vi "SCB RT.vi"() -> ()   [LabVIEW 2015]
uses:
  <vilib>/Platform/TimedLoop/XDataNode/XDataNode.xnode
  <vilib>/Platform/TimedLoop/XDataNode/nitl_modes.ctl
  <vilib>/Platform/TimedLoop/XDataNode/XDNodeRunTimeDep.lvlib
  <vilib>/Platform/TimedLoop/XDataNode/wakeup.ctl
  <vilib>/Platform/TimedLoop/XDataNode/timing_clust.ctl
  <vilib>/Platform/TimedLoop/XDataNode/loadnilvce.vi
  SC2 states.ctl
  <vilib>/Motion/BlockNode/FB.NIMotion.xnode
  <vilib>/nisyscfg/nisyscfg.lvlib
  Encoder bit cluster.ctl
  <vilib>/Motion/Express/_s/nimc.fb.straightLineMove.startStraightLineMove.axis.modeRelative.0.vi
  Horizontal Rod states.ctl
  GV states.ctl
  Vertical Rod states.ctl
  <vilib>/nisyscfg/Find Hardware.vi
  Bypass control.ctl
panel:
  out "SCB Wheel GV Bypass":bool
  out "SCB Sample Rod Bypass":bool
  out "SCB Retract Rod Bypass":bool
  out "SCB Ion Source GV Bypass":bool
  out "SCB Insert Rod Bypass":bool
  in  "Current State":T1
  out "Encoder displacement":i32
  in  "Random Sample":bool
  out "Within window?":bool
  in  "Stop":bool
  out "Motor status":bool=TRUE
  in  "Encoder offset":i32=-1277
  in  "Start Sample Change":bool
  out "SCB State Control":T1=enum."wait"
  out "Encoder readback":errorcluster
  in  "error in (no error)":errorcluster
  out "status":bool
  out "Encoder destination":i32
  in  "New Move (Motor steps)":dbl=10000.0 format="%#_13g"
  in  "New Sample":i16
  in  "Step Window radius":i32=2
  out "Converted Encoder":bool[](array[boolean])
  in  "Motion Resource":refnum<k21>="Axis SCB motor"
  out "Straight Line Move":errorcluster
  out "Raw Encoder":bool[](array[boolean])
  out "Encoder rotation":u16(graph)
  out "Encoder Position":i32
  # "Encoder offset required to \n\"line up\" encoder with wheel.\nSample 64 is -1021 encoder steps\n (or +15362 steps) from the \nencoder's zero point.. Note: Sample \nand encoder numbering run in \nopposite directions"
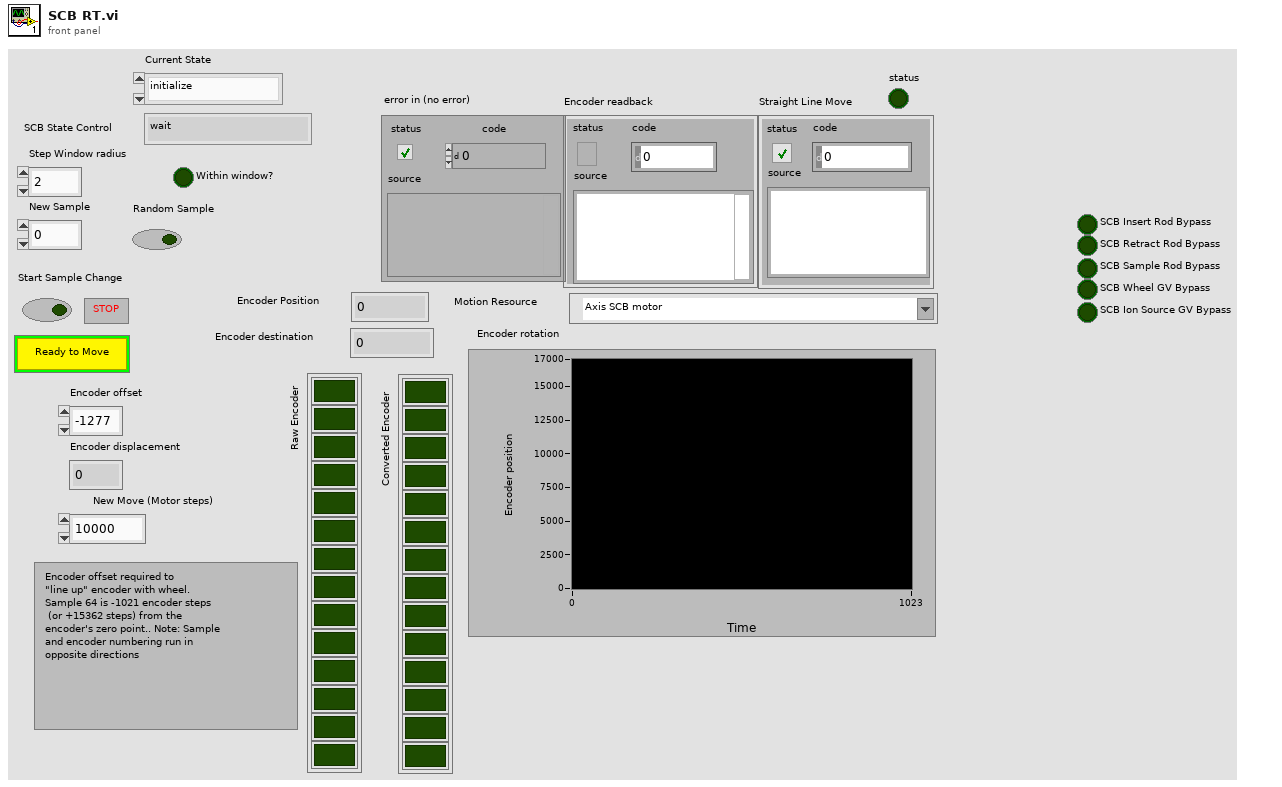
[diagram p1: front panel]
types:
  T1 = typedef "SC2 states.ctl" = enum16{"initialize", "wait", "change sample start", "change sample", "check position", "rotate wheel", "rotate complete", "sample rod up", "sample rod down", "retract rod in", "retract rod out", "insert rod in", "insert rod out", "bellows SC GV open", "bellows SC GV close", "bellows IS GV open", "bellows IS GV close", "vent source", "pump source", "rezero", "Shutdown"}
  T2 = typedef "XDNodeRunTimeDep.lvlib/timing_clust.ctl" = cluster{"Expected End [f-1]":u64, "Actual End [f-1]":u64, "Finished Late? [f-1]":bool, "Expected End [i-1]":u64, "Actual End [i-1]":u64, "Finished Late? [i-1]":bool, "Expected Start [i]":u64, "Actual Start [i]":u64, "Expected Start [f]":u64, "Actual Start [f]":u64, "Source Name":string, "Structure Name":string, "Period":i64, "Deadline":i64, "Offset":i64, "Start":i64, "Priority":i32, "Timeout":i32, "Mode":T3, "Wakeup Reason":T4, "Error":errorcluster, "Source Type":string, "Secondary Source Type":string, "Global End Time":u64, "Global Start Time":u64, "Frame Duration":u64, "Iteration Duration":u64, "Assigned CPU":i32, "I/O Scan Engine Mode":u32}
  T3 = typedef "XDNodeRunTimeDep.lvlib/nitl_modes.ctl" = enum32{"No Change", "Process missed periods, maintain original phase", "Discard missed periods, maintain original phase", "Process missed periods, ignore original phase", "Discard missed periods, ignore original phase"}
  T4 = typedef "XDNodeRunTimeDep.lvlib/wakeup.ctl" = enum32{"Normal", "Aborted", "Asynchronous wakeup", "Timing source error", "Timed loop error", "Timeout"}
  T5 = typedef "GV states.ctl" = enum16{"status unclear", "closed", "open"}
  T6 = typedef "Vertical Rod states.ctl" = enum16{"status unclear", "rod down", "rod up"}
  T7 = typedef "Horizontal Rod states.ctl" = enum16{"status unclear", "rod in", "rod out"}
  T8 = cluster{"Sample Rod":u16, "Insert Rod":u16, "Retract Rod":u16, "Wheel GV":u16, "Ion Source GV":u16, "Rotate Wheel":u16}
  T9 = typedef "Encoder bit cluster.ctl" = cluster{"MSB":bool, "13th bit":bool, "12th bit":bool, "11th bit":bool, "10th bit":bool, "9th bit":bool, "8th bit":bool, "7th bit":bool, "6th bit":bool, "5th bit":bool, "4th bit":bool, "3rd bit":bool, "2nd bit":bool, "LSB":bool}
  T10 = typedef "Bypass control.ctl" = cluster{"SCB Insert Rod Bypass":bool, "SCB Ion Source GV Bypass":bool, "SCB Retract Rod Bypass":bool, "SCB Sample Rod Bypass":bool, "SCB Wheel GV Bypass":bool}
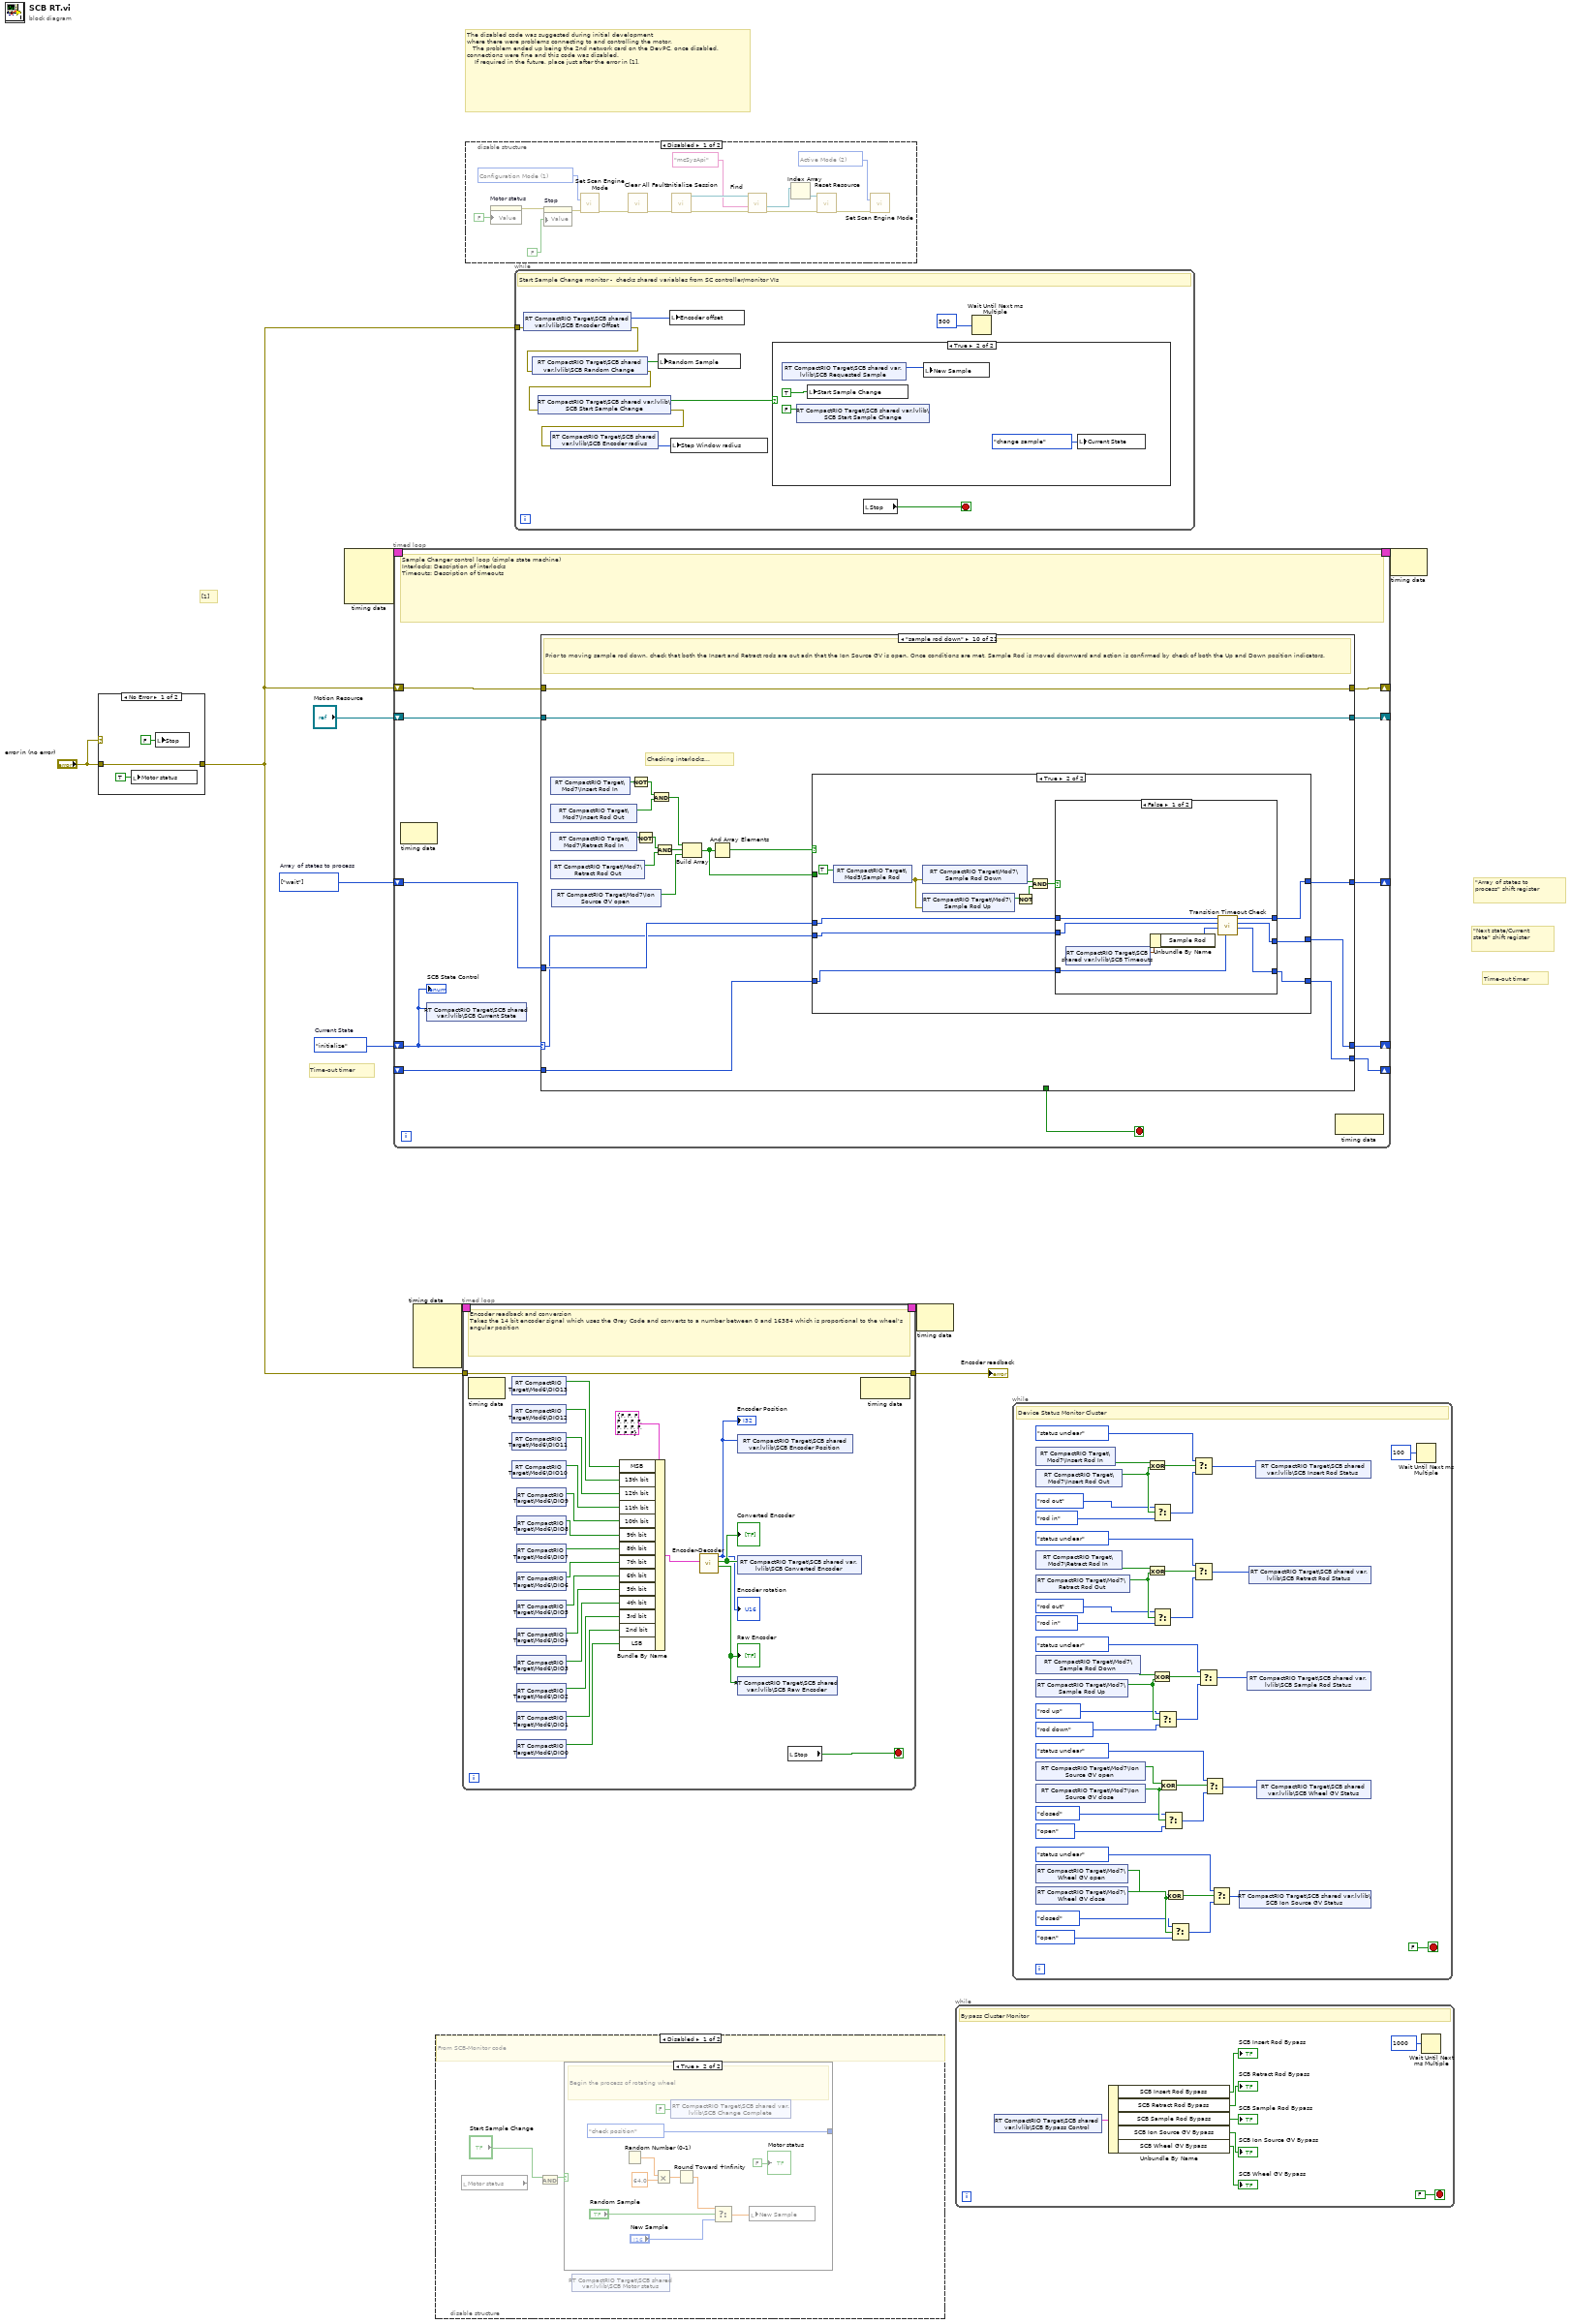
[diagram p0: block diagram]
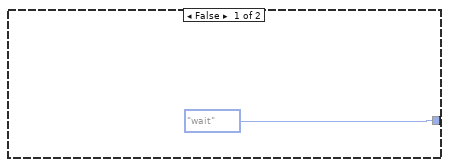
[diagram p2: hidden frame]
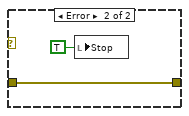
[diagram p4: hidden frame]
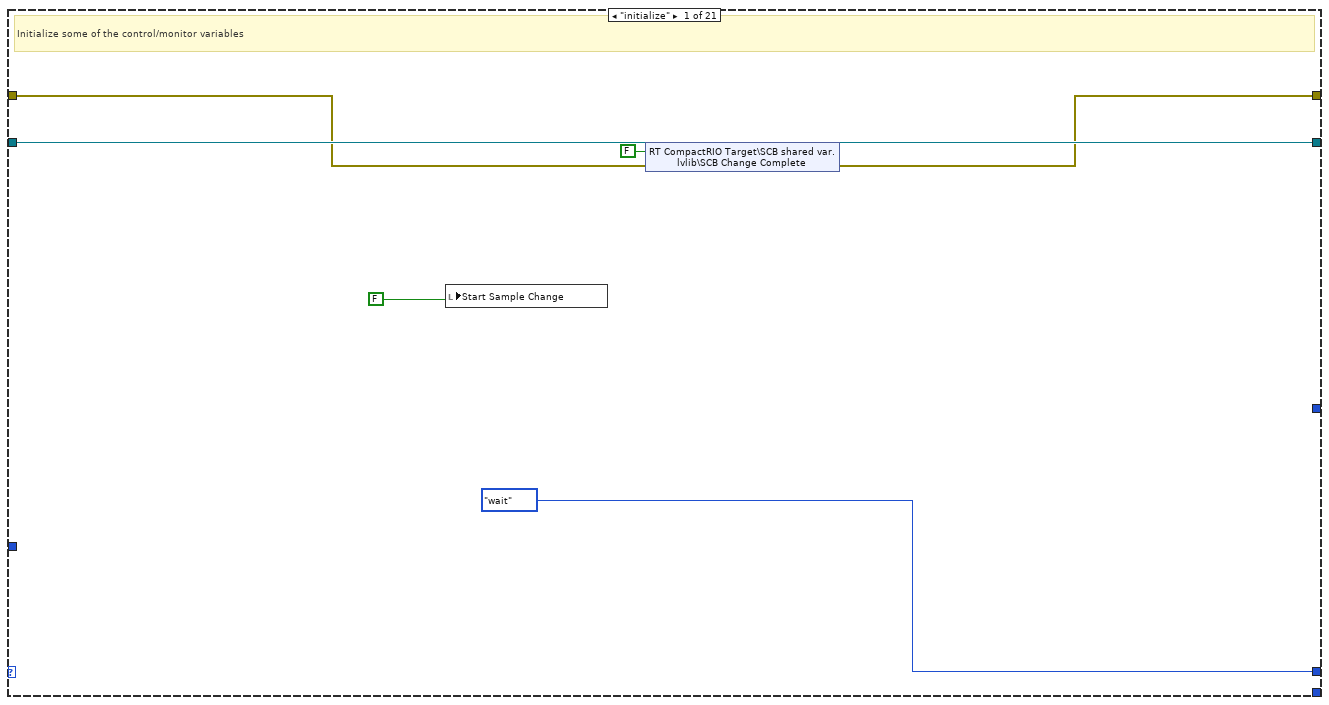
[diagram p7: hidden frame]
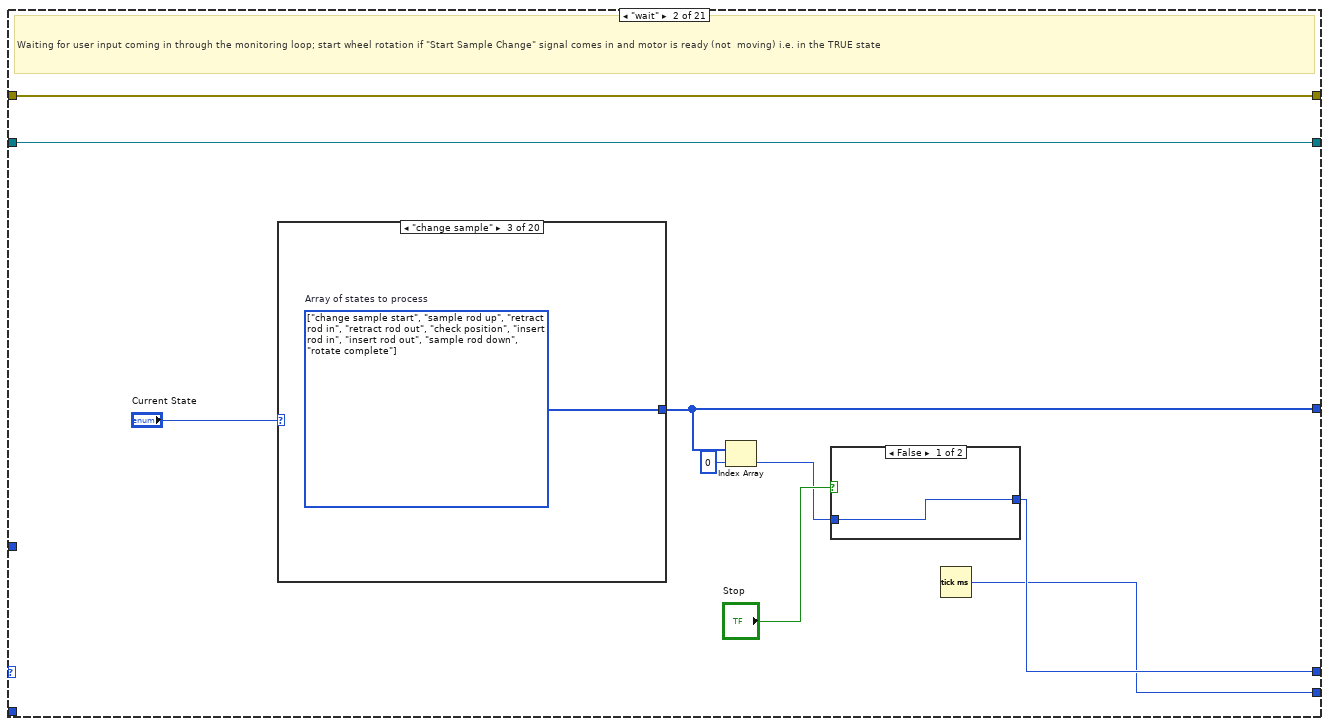
[diagram p8: hidden frame]
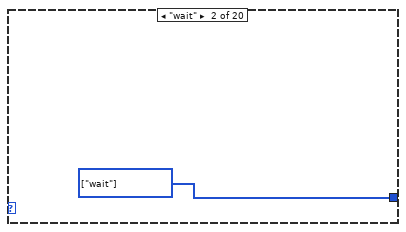
[diagram p10: hidden frame]
diagram:
  w1 = T1[] [enum."wait"] items=["initialize", "wait", "change sample start", "change sample", "check position", "rotate wheel", "rotate complete", "sample rod up", "sample rod down", "retract rod in", "retract rod out", "insert rod in", "insert rod out", "bellows SC GV open", "bellows SC GV close", "bellows IS GV open", "bellows IS GV close", "vent source", "pump source", "rezero", "Shutdown"]  # Array of states to process
  w5 = SC2_states."initialize"  # Current State
  # "Time-out timer"
  # "Time-out timer"
  # "\"Next state/Current\nstate\" shift register"
  # "\"Array of states to \nprocess\" shift register"
  # "[1]"
  # "The disabled code was suggested during initial development\nwhere there were problems connecting to and controlling the motor.\n   The problem ended up being the 2nd network card on the DevPC, once disabled, connections were fine and this code was disabled.  \n    If required in the future, place just after the error in [1]."
  n1 = case shown="No Error" "error in (no error)" {
    tunnel: "error in (no error)" -> [w12 w15]
    tunnel: [w12 w15] -> w3
    frame No Error {
      n2 = local write "Motor status"(TRUE ("Motor status")) -> ()
      n3 = local write "Stop"(FALSE ("Stop")) -> ()
    }
    frame Error {
      n4 = local write "Stop"(TRUE ("Stop")) -> ()
    }
  }
  n5 = node-c288() -> (w8:T2)  [unwired: 4 in]
  n6 = timed-loop {
    timing: w8 -> [_]
    timing-out: [_] -> w7
    shift-right: [w25] -> _
    shift-left: w5 -> [w22]
    shift-right: [w24] -> _
    shift-left: "Motion Resource" -> [w26]
    shift-right: [w20] -> _
    shift-left: w1 -> [w19]
    shift-right: [w18] -> _
    shift-left: _ -> [w17]
    shift-right: [w16] -> _
    shift-left: w3 -> [w23]
    stop <- w21 stop-if-true
    # "Sample Changer control loop (simple state machine)\nInterlocks: Description of interlocks\nTimeouts: Description of timeouts"
    n7 = node-c288() -> ()  [unwired: 1 in, 1 out]
    n8 = shared-variable "RT CompactRIO Target\\SCB shared var.lvlib\\SCB Current State"(w22) -> ()  [unwired: 1 in, 1 out]
    n9 = case shown="\"sample rod down\"" w22 {
      selector: w22 -> [_ _ w55 _ _ _ _ _ w140 w164 w229 w304 _ w335 _ w363 _ w421 _ _ _]
      tunnel: w26 -> [w31 w41 w46 w61 w89 w114 w134 _ _ w160 w240 _ _ w327 _ _ _ w416 _ _ _]
      tunnel: [SC2_states."wait" w39 w51 w74 w84 SC2_states."wait" SC2_states."Shutdown" _ w138 w165 w243 w300 _ w332 _ w361 _ w418 _ _ _] -> w25
      tunnel: [w31 w41 w46 w61 w81 w111 w134 _ _ w160 w240 _ _ w327 _ _ _ w416 _ _ _] -> w24
      tunnel: w23 -> [w28 w33 w49 w58 w78 _ _ _ _ w161 w241 _ _ w328 _ _ _ w415 _ _ _]
      tunnel: [_ _ _ _ _ _ TRUE _ _ _ _ _ _ _ _ _ _ _ _ _ _] -> w21
      tunnel: [_ w37 w54 _ w75 _ _ _ w139 w166 w244 w301 _ w333 _ w362 _ w417 _ _ _] -> w20
      tunnel: w19 -> [_ _ w56 _ w75 _ _ _ w141 w167 w228 w302 _ w336 _ w364 _ w422 _ _ _]
      tunnel: [_ w34 w50 w57 _ _ _ _ w137 w162 w242 w299 _ w331 _ w360 _ w419 _ _ _] -> w18
      tunnel: w17 -> [_ _ _ _ _ _ _ _ w136 w163 w245 w303 _ w334 _ w359 _ w420 _ _ _]
      tunnel: [w27 w33 w47 w58 w76 _ _ _ _ w161 w241 _ _ w328 _ _ _ w415 _ _ _] -> w16
      frame "initialize" {
        # "Initialize some of the control/monitor variables"
        n10 = local write "Start Sample Change"(FALSE ("Start Sample Change")) -> ()
        n11 = shared-variable "RT CompactRIO Target\\SCB shared var.lvlib\\SCB Change Complete"(FALSE ("SC2 Change Complete"), error in=w28) -> (error out=w27:errorcluster)
      }
      frame "wait" {
        # "Waiting for user input coming in through the monitoring loop; start wheel rotation if \"Start Sample Change\" signal comes in and motor is ready (not  moving) i.e. in the TRUE state"
        n12 = case shown="\"change sample\"" "Current State" {
          tunnel: [_ w42 w43 _ _ _ _ _ _ _ _ _ _ _ _ _ _ _ _ _] -> w37
          frame "initialize", Default {
          }
          frame "wait" {
            w42 = T1[] [enum."wait"] items=["initialize", "wait", "change sample start", "change sample", "check position", "rotate wheel", "rotate complete", "sample rod up", "sample rod down", "retract rod in", "retract rod out", "insert rod in", "insert rod out", "bellows SC GV open", "bellows SC GV close", "bellows IS GV open", "bellows IS GV close", "vent source", "pump source", "rezero", "Shutdown"] ("Array of states to process")
          }
          frame "change sample" {
            w43 = T1[] [enum."change sample start", enum."sample rod up", enum."retract rod in", enum."retract rod out", enum."check position", enum."insert rod in", enum."insert rod out", enum."sample rod down", enum."rotate complete"] items=["initialize", "wait", "change sample start", "change sample", "check position", "rotate wheel", "rotate complete", "sample rod up", "sample rod down", "retract rod in", "retract rod out", "insert rod in", "insert rod out", "bellows SC GV open", "bellows SC GV close", "bellows IS GV open", "bellows IS GV close", "vent source", "pump source", "rezero", "Shutdown"]  # Array of states to process
          }
          frame "check position" {
          }
          frame "rotate wheel" {
          }
          frame "rotate complete" {
          }
          frame "sample rod up" {
          }
          frame "sample rod down" {
          }
          frame "retract rod in" {
          }
          frame "retract rod out" {
          }
          frame "insert rod in" {
          }
          frame "insert rod out" {
          }
          frame "bellows SC GV open" {
          }
          frame "bellows SC GV close" {
          }
          frame "bellows IS GV open" {
          }
          frame "bellows IS GV close" {
          }
          frame "vent source" {
          }
          frame "pump source" {
          }
          frame "rezero" {
          }
          frame "Shutdown" {
          }
        }
        n13 = Index Array(array=w37, index=0) -> (element=w36:T1)
        n14 = case shown="False" "Stop" {
          tunnel: [w44 SC2_states."Shutdown"] -> w39
          tunnel: w36 -> [w44 _]
          frame False {
          }
          frame True {
          }
        }
        n15 = Tick Count (ms)() -> (millisecond timer value=w34:u32)
      }
      frame "change sample start" {
        n16 = call "Modify array of states.vi"("Current State"=w55, "Array of states to process"=w56) -> ("Next State"=w51:T1, "Modified Array of states"=w54:T1[])  [unwired: 8 in]
        n17 = shared-variable "RT CompactRIO Target\\SCB shared var.lvlib\\SCB Change Complete"(FALSE ("SCB Change Complete"), error in=w49) -> (error out=w48:errorcluster)
        n18 = shared-variable "RT CompactRIO Target\\SCB shared var.lvlib\\SCB Changing Sample"(TRUE ("SCB Changing Sample"), error in=w48) -> (error out=w47:errorcluster)
        n19 = Tick Count (ms)() -> (millisecond timer value=w50:u32)
      }
      frame "check position" {
        # "Number of steps for\nmotor to move"
        # "number of encoder steps to progress"
        # "14-bit encoder has 2^14 steps/rev"
        # "Motor steps per revolution"
        # "In this case, the wheel's position is checked and if it's within the Step WIndow Radius of the desired position, the state machine progresses to the \"rotate complete\" state.  If not, the number of encoder steps to progress to the desired position is stepped through by going to the \"rotate wheel\" state"
        n20 = local read "Encoder Position"() -> (w68:i32)
        n21 = local read "New Sample"() -> (w60:i16)
        n22 = call "Sample-Encoder conversion.vi"("Encoder Position"=w68, "Step Window radius"="Step Window radius", "New Sample Number"=w60, "Encoder offset"="Encoder offset") -> ("Encoder destination"=w66:i32, "Within Range?"=w59:bool, "Encoder displacement"=w69:i32)  [unwired: 5 in]
        "Encoder destination" <- w66
        "Within window?" <- w59
        "Encoder displacement" <- w69
        n23 = shared-variable "RT CompactRIO Target\\SCB shared var.lvlib\\SCB Encoder destination"(w66) -> ()  [unwired: 1 in, 1 out]
        n24 = Divide(x=50000.0, y=16384.0) -> (x/y=w73:dbl)
        n25 = Multiply(x=w73, y=w69) -> (x*y=w70:dbl)
        n26 = local write "Motor status"(w59) -> ()
        n27 = shared-variable "RT CompactRIO Target\\SCB shared var.lvlib\\SCB Motor status"(w59) -> ()  [unwired: 1 in, 1 out]
        n28 = Round To Nearest(number=w70) -> (nearest integer value=w63:dbl)
        n29 = local write "New Move (Motor steps)"(w63) -> ()
        n30 = Select(t=SC2_states."rotate complete", s=w59, f=SC2_states."rotate wheel") -> (s? t:f=w74:T1)
        n31 = Tick Count (ms)() -> (millisecond timer value=w57:u32)
      }
      frame "rotate wheel" {
        w90 = 10000.0
        # "Prior to Rotating Wheel, both Insert and Retract rods' positions are checked.  Once confirmed, step motor to progress though New Move number of steps and then returns to \"check position\" to determine that the move was successful"
        n32 = local read "Start Sample Change"() -> (w85:bool)
        n33 = Multiply(x="New Move (Motor steps)", y=-1.0) -> (x*y=w80:dbl)
        n34 = xnode "Straight-Line Move\n(Relative)"("error in"=w78, "resource"=w89, "execute"=w85, "position"=w80, "velocity"=w90, "acceleration"=w90) -> ("error out"=w76:errorcluster, "resource out"=w81:refnum<k21>, "done"=w82:bool)
        "Straight Line Move" <- w76
        n35 = Unbundle By Name(w76) -> ("status"=→"status":bool)
        n36 = Not(x=w82) -> (.not. x?=w77:bool)
        n37 = local write "Start Sample Change"(w77) -> ()
        n38 = Select(t=SC2_states."check position", s=w82, f=SC2_states."rotate wheel") -> (s? t:f=w84:T1)
      }
      frame "rotate complete" {
        # "Stop SLM; set monitor variables"
        n39 = local read "New Sample"() -> (w109:i16)
        n40 = xnode "Straight-Line Move\n(Relative)"("resource"=w114, "execute"=FALSE) -> ("resource out"=w111:refnum<k21>)  [unwired: 4 in, 2 out]
        n41 = shared-variable "RT CompactRIO Target\\SCB shared var.lvlib\\SCB Current Sample"(w109) -> ()  [unwired: 1 in, 1 out]
        n42 = shared-variable "RT CompactRIO Target\\SCB shared var.lvlib\\SCB Change Complete"(TRUE ("SC2 Change Complete")) -> ()  [unwired: 1 in, 1 out]
        n43 = local write "Start Sample Change"(FALSE ("Start Sample Change")) -> ()
      }
      frame "Shutdown" {
      }
      frame "change sample" {
      }
      frame "sample rod up" {
        # "Move Sample Rod upward; check both the up and down position indicators"
        n44 = shared-variable "RT CompactRIO Target\\Mod5\\Sample Rod"(FALSE) -> (error out=w135:errorcluster)  [unwired: 1 in]
        n45 = shared-variable "RT CompactRIO Target\\Mod7\\Sample Rod Up"(error in=w135) -> (w143:bool)  [unwired: 1 out]
        n46 = shared-variable "RT CompactRIO Target\\Mod7\\Sample Rod Down"(error in=w135) -> (w145:bool)  [unwired: 1 out]
        n47 = Not(x=w145) -> (.not. x?=w144:bool)
        n48 = And(x=w143, y=w144) -> (x .and. y?=w142:bool)
        n49 = case shown="True" w142 {
          tunnel: w141 -> [w152 w159]
          tunnel: w140 -> [w154 w158]
          tunnel: [w151 w157] -> w139
          tunnel: [w153 w156] -> w138
          tunnel: [w149 w155] -> w137
          tunnel: w136 -> [w150 _]
          frame False {
            # "Sample rod is not up. Check to see if timeout limit has been reached"
            n50 = shared-variable "RT CompactRIO Target\\SCB shared var.lvlib\\SCB Timeouts"() -> (w148:T8)  [unwired: 1 in, 1 out]
            n51 = Unbundle By Name(w148) -> ("Sample Rod"=w147:u16)
            n52 = call "Transition Timeout Check.vi"("Start Time"=w150, "Timeout limit"=w147, "Current State in"=w154, "Modified Array of states in"=w152) -> ("millisecond timer value out"=w149:u32, "Next State"=w153:T1, "Modified Array of states out"=w151:T1[])  [unwired: 4 in, 1 out]
          }
          frame True {
            # "Sample Rod is up; progress to next state and reset timer."
            n53 = call "Modify array of states.vi"("Current State"=w158, "Array of states to process"=w159) -> ("Next State"=w156:T1, "Modified Array of states"=w157:T1[])  [unwired: 8 in]
            n54 = Tick Count (ms)() -> (millisecond timer value=w155:u32)
          }
        }
      }
      frame "sample rod down" {
        # "Checking interlocks..."
        # "Prior to moving sample rod down, check that both the Insert and Retract rods are out adn that the Ion Source GV is open. Once conditions are met, Sample Rod is moved downward and action is confirmed by check of both the Up and Down position indicators."
        n55 = shared-variable "RT CompactRIO Target\\Mod7\\Insert Rod In"() -> (w178:bool)  [unwired: 1 in, 1 out]
        n56 = shared-variable "RT CompactRIO Target\\Mod7\\Insert Rod Out"() -> (w175:bool)  [unwired: 1 in, 1 out]
        n57 = shared-variable "RT CompactRIO Target\\Mod7\\Retract Rod In"() -> (w177:bool)  [unwired: 1 in, 1 out]
        n58 = shared-variable "RT CompactRIO Target\\Mod7\\Retract Rod Out"() -> (w173:bool)  [unwired: 1 in, 1 out]
        n59 = shared-variable "RT CompactRIO Target\\Mod7\\Ion Source GV open"() -> (w171:bool)  [unwired: 1 in, 1 out]
        n60 = Not(x=w178) -> (.not. x?=w176:bool)
        n61 = Not(x=w177) -> (.not. x?=w174:bool)
        n62 = And(x=w176, y=w175) -> (x .and. y?=w170:bool)
        n63 = And(x=w174, y=w173) -> (x .and. y?=w172:bool)
        n64 = Build Array(w170, w172, w171) -> (w168:bool[])
        n65 = And Array Elements(Boolean array=w168) -> (logical AND=w169:bool)
        n66 = case shown="True" w169 {
          tunnel: w168 -> [w185 _]
          tunnel: w167 -> [w182 w203]
          tunnel: [w181 w200] -> w166
          tunnel: [w180 w199] -> w165
          tunnel: w164 -> [_ w202]
          tunnel: w163 -> [_ w201]
          tunnel: [w179 w198] -> w162
          frame False {
            n67 = Search 1D Array(1D array=w185, element=FALSE) -> (index of element=w183:i32)  [unwired: 1 in]
            n68 = case shown="2" w183 {
              tunnel: w182 -> [w188 w190 w196]
              tunnel: [w187 w191 w194] -> w181
              tunnel: [w186 w192 w195] -> w180
              frame 0, Default {
                w186 = SC2_states."insert rod out"
                # "Insert Rod not completely out"
                n69 = Insert Into Array(array=w188, index=0, new element=w186) -> (w187:T1[])
              }
              frame 1 {
                w192 = SC2_states."retract rod out"
                # "Retract Rod not completely out"
                n70 = Insert Into Array(array=w190, index=0, new element=w192) -> (w191:T1[])
              }
              frame 2 {
                w195 = SC2_states."bellows IS GV open"
                # "Ion Source GV is still closed"
                n71 = Insert Into Array(array=w196, index=0, new element=w195) -> (w194:T1[])
              }
            }
            n72 = Tick Count (ms)() -> (millisecond timer value=w179:u32)
          }
          frame True {
            n73 = shared-variable "RT CompactRIO Target\\Mod5\\Sample Rod"(TRUE ("Wheel GV")) -> (error out=w208:errorcluster)  [unwired: 1 in]
            n74 = shared-variable "RT CompactRIO Target\\Mod7\\Sample Rod Down"(error in=w208) -> (w205:bool)  [unwired: 1 out]
            n75 = shared-variable "RT CompactRIO Target\\Mod7\\Sample Rod Up"(error in=w208) -> (w207:bool)  [unwired: 1 out]
            n76 = Not(x=w207) -> (.not. x?=w206:bool)
            n77 = And(x=w205, y=w206) -> (x .and. y?=w204:bool)
            n78 = case shown="False" w204 {
              tunnel: w203 -> [w216 w222]
              tunnel: w202 -> [w215 w221]
              tunnel: [w210 w220] -> w200
              tunnel: [w211 w219] -> w199
              tunnel: [w212 w218] -> w198
              tunnel: w201 -> [w213 _]
              frame False {
                n79 = shared-variable "RT CompactRIO Target\\SCB shared var.lvlib\\SCB Timeouts"() -> (w217:T8)  [unwired: 1 in, 1 out]
                n80 = Unbundle By Name(w217) -> ("Sample Rod"=w214:u16)
                n81 = call "Transition Timeout Check.vi"("Start Time"=w213, "Timeout limit"=w214, "Current State in"=w215, "Modified Array of states in"=w216) -> ("millisecond timer value out"=w212:u32, "Next State"=w211:T1, "Modified Array of states out"=w210:T1[])  [unwired: 4 in, 1 out]
              }
              frame True {
                n82 = call "Modify array of states.vi"("Current State"=w221, "Array of states to process"=w222) -> ("Next State"=w219:T1, "Modified Array of states"=w220:T1[])  [unwired: 8 in]
                n83 = Tick Count (ms)() -> (millisecond timer value=w218:u32)
              }
            }
          }
        }
      }
      frame "retract rod in" {
        # "Checking interlocks..."
        # "Prior to moving Retract Rod inward, check that: (1) the Sample Rod is UP; (2) the Insert Rod is OUT; and (3) the Wheel GV is open. Once conditions are met, Retract Rod is moved inward and action is confirmed by check of both the IN and OUT position indicators."
        n84 = local read "SCB Insert Rod Bypass"() -> (w236:bool)
        n85 = shared-variable "RT CompactRIO Target\\SCB shared var.lvlib\\SCB Insert Rod Status"() -> (w238:T7)  [unwired: 1 in, 1 out]
        n86 = local read "SCB Sample Rod Bypass"() -> (w232:bool)
        n87 = shared-variable "RT CompactRIO Target\\SCB shared var.lvlib\\SCB Sample Rod Status"() -> (w231:T6)  [unwired: 1 in, 1 out]
        n88 = local read "SCB Wheel GV Bypass"() -> (w226:bool)
        n89 = shared-variable "RT CompactRIO Target\\SCB shared var.lvlib\\SCB Wheel GV Status"() -> (w224:T5)  [unwired: 1 in, 1 out]
        n90 = Equal?(x=w224, y=GV_states."open") -> (x = y?=w225:bool)
        n91 = Equal?(x=w231, y=Vertical_Rod_states."rod up") -> (x = y?=w233:bool)
        n92 = Equal?(x=w238, y=Horizontal_Rod_states."rod out") -> (x = y?=w237:bool)
        n93 = Or(x=w226, y=w225) -> (x .or. y?=w227:bool)
        n94 = Or(x=w232, y=w233) -> (x .or. y?=w234:bool)
        n95 = Or(x=w236, y=w237) -> (x .or. y?=w235:bool)
        n96 = Build Array(w235, w234, w227) -> (w246:bool[])
        n97 = And Array Elements(Boolean array=w246) -> (logical AND=w247:bool)
        n98 = case shown="False" w247 {
          tunnel: w246 -> [w254 _]
          tunnel: w228 -> [w251 w274]
          tunnel: [w250 w271] -> w244
          tunnel: [w249 w270] -> w243
          tunnel: w229 -> [_ w273]
          tunnel: w245 -> [_ w272]
          tunnel: [w248 w269] -> w242
          frame False {
            n99 = Search 1D Array(1D array=w254, element=FALSE) -> (index of element=w252:i32)  [unwired: 1 in]
            n100 = case shown="1" w252 {
              tunnel: w251 -> [w257 w259 w265]
              tunnel: [w256 w260 w263] -> w250
              tunnel: [w255 w261 w264] -> w249
              frame 0, Default {
                w255 = SC2_states."insert rod out"
                # "Insert Rod not completely out"
                n101 = Insert Into Array(array=w257, index=0, new element=w255) -> (w256:T1[])
              }
              frame 1 {
                w261 = SC2_states."sample rod up"
                # "Sample Rod not completely up"
                n102 = Insert Into Array(array=w259, index=0, new element=w261) -> (w260:T1[])
              }
              frame 2 {
                w264 = SC2_states."bellows SC GV open"
                # "Wheel GV is still closed"
                n103 = Insert Into Array(array=w265, index=0, new element=w264) -> (w263:T1[])
              }
            }
            n104 = Tick Count (ms)() -> (millisecond timer value=w248:u32)
          }
          frame True {
            n105 = shared-variable "RT CompactRIO Target\\Mod5\\Retract Rod"(TRUE ("Wheel GV")) -> (error out=w267:errorcluster)  [unwired: 1 in]
            n106 = shared-variable "RT CompactRIO Target\\SCB shared var.lvlib\\SCB Retract Rod Status"(error in=w267) -> (w268:T7)  [unwired: 1 out]
            n107 = case shown="\"rod in\"" w268 {
              tunnel: w274 -> [w282 w290 w296]
              tunnel: w273 -> [w281 w289 w295]
              tunnel: [w276 w284 w294] -> w271
              tunnel: [w277 w285 w293] -> w270
              tunnel: [w278 w286 w292] -> w269
              tunnel: w272 -> [w279 w287 _]
              frame "status unclear", Default {
                n108 = shared-variable "RT CompactRIO Target\\SCB shared var.lvlib\\SCB Timeouts"() -> (w283:T8)  [unwired: 1 in, 1 out]
                n109 = Unbundle By Name(w283) -> ("Retract Rod"=w280:u16)
                n110 = call "Transition Timeout Check.vi"("Start Time"=w279, "Timeout limit"=w280, "Current State in"=w281, "Modified Array of states in"=w282) -> ("millisecond timer value out"=w278:u32, "Next State"=w277:T1, "Modified Array of states out"=w276:T1[])  [unwired: 4 in, 1 out]
              }
              frame "rod out" {
                n111 = shared-variable "RT CompactRIO Target\\SCB shared var.lvlib\\SCB Timeouts"() -> (w291:T8)  [unwired: 1 in, 1 out]
                n112 = Unbundle By Name(w291) -> ("Retract Rod"=w288:u16)
                n113 = call "Transition Timeout Check.vi"("Start Time"=w287, "Timeout limit"=w288, "Current State in"=w289, "Modified Array of states in"=w290) -> ("millisecond timer value out"=w286:u32, "Next State"=w285:T1, "Modified Array of states out"=w284:T1[])  [unwired: 4 in, 1 out]
              }
              frame "rod in" {
                n114 = call "Modify array of states.vi"("Current State"=w295, "Array of states to process"=w296) -> ("Next State"=w293:T1, "Modified Array of states"=w294:T1[])  [unwired: 8 in]
                n115 = Tick Count (ms)() -> (millisecond timer value=w292:u32)
              }
            }
          }
        }
      }
      frame "retract rod out" {
        # "Move Retract Rod outward; check both the in and out position indicators"
        n116 = shared-variable "RT CompactRIO Target\\Mod5\\Retract Rod"(FALSE) -> (error out=w298:errorcluster)  [unwired: 1 in]
        n117 = shared-variable "RT CompactRIO Target\\SCB shared var.lvlib\\SCB Retract Rod Status"(error in=w298) -> (w297:T7)  [unwired: 1 out]
        n118 = case shown="\"rod out\"" w297 {
          tunnel: w302 -> [w311 w318 w324]
          tunnel: w304 -> [w313 w317 w326]
          tunnel: [w310 w316 w323] -> w301
          tunnel: [w312 w315 w325] -> w300
          tunnel: [w308 w314 w321] -> w299
          tunnel: w303 -> [w309 _ w322]
          frame "status unclear", Default {
            # "Retract rod is not out. Check to see if timeout limit has been reached"
            n119 = shared-variable "RT CompactRIO Target\\SCB shared var.lvlib\\SCB Timeouts"() -> (w307:T8)  [unwired: 1 in, 1 out]
            n120 = Unbundle By Name(w307) -> ("Retract Rod"=w306:u16)
            n121 = call "Transition Timeout Check.vi"("Start Time"=w309, "Timeout limit"=w306, "Current State in"=w313, "Modified Array of states in"=w311) -> ("millisecond timer value out"=w308:u32, "Next State"=w312:T1, "Modified Array of states out"=w310:T1[])  [unwired: 4 in, 1 out]
          }
          frame "rod out" {
            # "Retract Rod is out; progress to next state and reset timer."
            n122 = call "Modify array of states.vi"("Current State"=w317, "Array of states to process"=w318) -> ("Next State"=w315:T1, "Modified Array of states"=w316:T1[])  [unwired: 8 in]
            n123 = Tick Count (ms)() -> (millisecond timer value=w314:u32)
          }
          frame "rod in" {
            # "Retract rod is not out. Check to see if timeout limit has been reached"
            n124 = shared-variable "RT CompactRIO Target\\SCB shared var.lvlib\\SCB Timeouts"() -> (w320:T8)  [unwired: 1 in, 1 out]
            n125 = Unbundle By Name(w320) -> ("Retract Rod"=w319:u16)
            n126 = call "Transition Timeout Check.vi"("Start Time"=w322, "Timeout limit"=w319, "Current State in"=w326, "Modified Array of states in"=w324) -> ("millisecond timer value out"=w321:u32, "Next State"=w325:T1, "Modified Array of states out"=w323:T1[])  [unwired: 4 in, 1 out]
          }
        }
      }
      frame "insert rod in" {
        # "Prior to moving Insert Rod inward, check that: (1) the Sample Rod is UP; (2) the Retract Rod is OUT; and (3) the Wheel GV is open. Once conditions are met, Insert Rod is moved inward and action is confirmed by check of both the IN and OUT position indicators."
      }
      frame "insert rod out" {
        # "Move Insert Rod outward; check both the in and out position indicators"
        n127 = shared-variable "RT CompactRIO Target\\Mod5\\Insert Rod"(FALSE) -> (error out=w329:errorcluster)  [unwired: 1 in]
        n128 = shared-variable "RT CompactRIO Target\\SCB shared var.lvlib\\SCB Insert Rod Status"(error in=w329) -> (w330:T7)  [unwired: 1 out]
        n129 = case shown="\"rod out\"" w330 {
          tunnel: w336 -> [w343 w350 w356]
          tunnel: w335 -> [w345 w349 w358]
          tunnel: [w342 w348 w355] -> w333
          tunnel: [w344 w347 w357] -> w332
          tunnel: [w340 w346 w353] -> w331
          tunnel: w334 -> [w341 _ w354]
          frame "status unclear", Default {
            # "Insert Rod is not out. Check to see if timeout limit has been reached"
            n130 = shared-variable "RT CompactRIO Target\\SCB shared var.lvlib\\SCB Timeouts"() -> (w339:T8)  [unwired: 1 in, 1 out]
            n131 = Unbundle By Name(w339) -> ("Insert Rod"=w338:u16)
            n132 = call "Transition Timeout Check.vi"("Start Time"=w341, "Timeout limit"=w338, "Current State in"=w345, "Modified Array of states in"=w343) -> ("millisecond timer value out"=w340:u32, "Next State"=w344:T1, "Modified Array of states out"=w342:T1[])  [unwired: 4 in, 1 out]
          }
          frame "rod out" {
            # "Insert Rod is out; progress to next state and reset timer."
            n133 = call "Modify array of states.vi"("Current State"=w349, "Array of states to process"=w350) -> ("Next State"=w347:T1, "Modified Array of states"=w348:T1[])  [unwired: 8 in]
            n134 = Tick Count (ms)() -> (millisecond timer value=w346:u32)
          }
          frame "rod in" {
            # "Insert Rod is not out. Check to see if timeout limit has been reached"
            n135 = shared-variable "RT CompactRIO Target\\SCB shared var.lvlib\\SCB Timeouts"() -> (w352:T8)  [unwired: 1 in, 1 out]
            n136 = Unbundle By Name(w352) -> ("Insert Rod"=w351:u16)
            n137 = call "Transition Timeout Check.vi"("Start Time"=w354, "Timeout limit"=w351, "Current State in"=w358, "Modified Array of states in"=w356) -> ("millisecond timer value out"=w353:u32, "Next State"=w357:T1, "Modified Array of states out"=w355:T1[])  [unwired: 4 in, 1 out]
          }
        }
      }
      frame "bellows SC GV open" {
      }
      frame "bellows SC GV close" {
        # "Checking interlocks..."
        # "Prior to closing Wheel GV, the Insert and Retract rods are confirmed to be OUT."
        n138 = shared-variable "RT CompactRIO Target\\Mod7\\Insert Rod In"() -> (w373:bool)  [unwired: 1 in, 1 out]
        n139 = shared-variable "RT CompactRIO Target\\Mod7\\Insert Rod Out"() -> (w371:bool)  [unwired: 1 in, 1 out]
        n140 = shared-variable "RT CompactRIO Target\\Mod7\\Retract Rod Out"() -> (w369:bool)  [unwired: 1 in, 1 out]
        n141 = shared-variable "RT CompactRIO Target\\Mod7\\Retract Rod In"() -> (w374:bool)  [unwired: 1 in, 1 out]
        n142 = Not(x=w373) -> (.not. x?=w372:bool)
        n143 = Not(x=w374) -> (.not. x?=w370:bool)
        n144 = And(x=w371, y=w372) -> (x .and. y?=w368:bool)
        n145 = And(x=w369, y=w370) -> (x .and. y?=w367:bool)
        n146 = Build Array(w368, w367) -> (w365:bool[])
        n147 = And Array Elements(Boolean array=w365) -> (logical AND=w366:bool)
        n148 = case shown="True" w366 {
          tunnel: w365 -> [w381 _]
          tunnel: w364 -> [w376 w395]
          tunnel: w363 -> [_ w394]
          tunnel: [w375 w393] -> w362
          tunnel: [w377 w392] -> w361
          tunnel: [w378 w391] -> w360
          tunnel: w359 -> [_ w390]
          frame False {
            n149 = Search 1D Array(1D array=w381, element=FALSE) -> (index of element=w379:i32)  [unwired: 1 in]
            n150 = case shown="0, Default" w379 {
              tunnel: [w382 w389] -> w377
              tunnel: w376 -> [w384 w387]
              tunnel: [w383 w386] -> w375
              frame 0, Default {
                w382 = SC2_states."insert rod out"
                # "Insert rod not completely out"
                n151 = Insert Into Array(array=w384, index=0, new element=w382) -> (w383:T1[])
              }
              frame 1 {
                w389 = SC2_states."retract rod out"
                # "Retract Rod not completely out"
                n152 = Insert Into Array(array=w387, index=0, new element=w389) -> (w386:T1[])
              }
            }
            n153 = Tick Count (ms)() -> (millisecond timer value=w378:u32)
          }
          frame True {
            n154 = shared-variable "RT CompactRIO Target\\Mod5\\Wheel GV"(FALSE ("Wheel GV")) -> (error out=w400:errorcluster)  [unwired: 1 in]
            n155 = shared-variable "RT CompactRIO Target\\Mod7\\Wheel GV open"(error in=w400) -> (w397:bool)  [unwired: 1 out]
            n156 = shared-variable "RT CompactRIO Target\\Mod7\\Wheel GV close"(error in=w400) -> (w399:bool)  [unwired: 1 out]
            n157 = Not(x=w399) -> (.not. x?=w398:bool)
            n158 = And(x=w397, y=w398) -> (x .and. y?=w396:bool)
            n159 = case shown="False" w396 {
              tunnel: w395 -> [w408 w414]
              tunnel: w394 -> [w407 w413]
              tunnel: [w402 w412] -> w393
              tunnel: [w403 w411] -> w392
              tunnel: [w404 w410] -> w391
              tunnel: w390 -> [w405 _]
              frame False {
                n160 = shared-variable "RT CompactRIO Target\\SCB shared var.lvlib\\SCB Timeouts"() -> (w409:T8)  [unwired: 1 in, 1 out]
                n161 = Unbundle By Name(w409) -> ("Wheel GV"=w406:u16)
                n162 = call "Transition Timeout Check.vi"("Start Time"=w405, "Timeout limit"=w406, "Current State in"=w407, "Modified Array of states in"=w408) -> ("millisecond timer value out"=w404:u32, "Next State"=w403:T1, "Modified Array of states out"=w402:T1[])  [unwired: 4 in, 1 out]
              }
              frame True {
                n163 = call "Modify array of states.vi"("Current State"=w413, "Array of states to process"=w414) -> ("Next State"=w411:T1, "Modified Array of states"=w412:T1[])  [unwired: 8 in]
                n164 = Tick Count (ms)() -> (millisecond timer value=w410:u32)
              }
            }
          }
        }
      }
      frame "bellows IS GV open" {
      }
      frame "bellows IS GV close" {
        # "Checking interlocks..."
        # "Prior to closing Ion Source GV, the Sample Rod is confirmed to be UP."
        n165 = shared-variable "RT CompactRIO Target\\Mod7\\Sample Rod Down"() -> (w426:bool)  [unwired: 1 in, 1 out]
        n166 = shared-variable "RT CompactRIO Target\\Mod7\\Sample Rod Up"() -> (w424:bool)  [unwired: 1 in, 1 out]
        n167 = Not(x=w426) -> (.not. x?=w425:bool)
        n168 = And(x=w424, y=w425) -> (x .and. y?=w423:bool)
        n169 = case shown="False" w423 {
          tunnel: w422 -> [w431 w437]
          tunnel: w421 -> [_ w436]
          tunnel: w420 -> [_ w435]
          tunnel: [w427 w434] -> w419
          tunnel: [w429 w433] -> w418
          tunnel: [w428 w432] -> w417
          frame False {
            w429 = SC2_states."sample rod up"
            n170 = Insert Into Array(array=w431, index=0, new element=w429) -> (w428:T1[])
            n171 = Tick Count (ms)() -> (millisecond timer value=w427:u32)
          }
          frame True {
            n172 = shared-variable "RT CompactRIO Target\\Mod5\\Ion Source GV"(FALSE ("Ion Source GV")) -> (error out=w442:errorcluster)  [unwired: 1 in]
            n173 = shared-variable "RT CompactRIO Target\\Mod7\\Ion Source GV close"(error in=w442) -> (w439:bool)  [unwired: 1 out]
            n174 = shared-variable "RT CompactRIO Target\\Mod7\\Ion Source GV open"() -> (w441:bool)  [unwired: 1 in, 1 out]
            n175 = Not(x=w441) -> (.not. x?=w440:bool)
            n176 = And(x=w439, y=w440) -> (x .and. y?=w438:bool)
            n177 = case shown="False" w438 {
              tunnel: w437 -> [w449 w456]
              tunnel: w436 -> [w451 w455]
              tunnel: [w448 w454] -> w432
              tunnel: [w450 w453] -> w433
              tunnel: [w446 w452] -> w434
              tunnel: w435 -> [w447 _]
              frame False {
                # "Timeout check"
                # "Ion Source GV is not closed. Check to see if timeout limit has been reached"
                n178 = shared-variable "RT CompactRIO Target\\SCB shared var.lvlib\\SCB Timeouts"() -> (w445:T8)  [unwired: 1 in, 1 out]
                n179 = Unbundle By Name(w445) -> ("Ion Source GV"=w444:u16)
                n180 = call "Transition Timeout Check.vi"("Start Time"=w447, "Timeout limit"=w444, "Current State in"=w451, "Modified Array of states in"=w449) -> ("millisecond timer value out"=w446:u32, "Next State"=w450:T1, "Modified Array of states out"=w448:T1[])  [unwired: 4 in, 1 out]
              }
              frame True {
                # "Ion Source GV is closed; progress to next state and reset timer."
                n181 = call "Modify array of states.vi"("Current State"=w455, "Array of states to process"=w456) -> ("Next State"=w453:T1, "Modified Array of states"=w454:T1[])  [unwired: 8 in]
                n182 = Tick Count (ms)() -> (millisecond timer value=w452:u32)
              }
            }
          }
        }
      }
      frame "vent source" {
      }
      frame "pump source" {
      }
      frame "rezero" {
      }
    }
    n183 = node-c288() -> ()  [unwired: 1 in, 1 out]
    "SCB State Control" <- w22
  }
  n184 = node-c288() -> (w10:T2)  [unwired: 5 in]
  n185 = disable-structure shown="Disabled" {
    frame Disabled {
      # "From SCB-Monitor code"
      n186 = local read "Motor status"() -> ()  [unwired: 1 out]
      n187 = And(x="Start Sample Change") -> (x .and. y?=w460:bool)  [unwired: 1 in]
      n188 = case shown="True" w460 {
        tunnel: [SC2_states."wait" SC2_states."check position"] -> _
        frame False {
        }
        frame True {
          # "Begin the process of rotating wheel"
          n189 = Random Number (0-1)() -> (number: 0 to 1=w470:dbl)
          n190 = Multiply(x=w470, y=64.0) -> (x*y=w471:dbl)
          n191 = shared-variable "RT CompactRIO Target\\SCB shared var.lvlib\\SCB Change Complete"(FALSE) -> ()  [unwired: 1 in, 1 out]
          n192 = Round Toward +Infinity(x=w471) -> (ceil(x): smallest int >= x=w465:dbl)
          n193 = Select(t=w465, s="Random Sample", f="New Sample") -> (s? t:f=w464:dbl)
          n194 = local write "New Sample"(w464) -> ()
          "Motor status" <- FALSE ("Motor status")
        }
      }
      n195 = shared-variable "RT CompactRIO Target\\SCB shared var.lvlib\\SCB Motor status"() -> ()  [unwired: 2 in, 1 out]
    }
    frame Enabled {
    }
  }
  n196 = timed-loop {
    timing: w10 -> [_]
    timing-out: [_] -> w9
    tunnel: w3 -> [w489]
    tunnel: [w489] -> w4
    stop <- w472 stop-if-true
    # "Encoder readback and conversion\nTakes the 14 bit encoder signal which uses the Grey Code and converts to a number between 0 and 16384 which is proportional to the wheel's angular position"
    n197 = node-c288() -> ()  [unwired: 1 in, 1 out]
    n198 = shared-variable "RT CompactRIO Target\\Mod6\\DIO13"() -> (w488:bool)  [unwired: 1 in, 1 out]
    n199 = shared-variable "RT CompactRIO Target\\Mod6\\DIO12"() -> (w487:bool)  [unwired: 1 in, 1 out]
    n200 = shared-variable "RT CompactRIO Target\\Mod6\\DIO11"() -> (w486:bool)  [unwired: 1 in, 1 out]
    n201 = shared-variable "RT CompactRIO Target\\Mod6\\DIO10"() -> (w485:bool)  [unwired: 1 in, 1 out]
    n202 = shared-variable "RT CompactRIO Target\\Mod6\\DIO9"() -> (w484:bool)  [unwired: 1 in, 1 out]
    n203 = shared-variable "RT CompactRIO Target\\Mod6\\DIO8"() -> (w483:bool)  [unwired: 1 in, 1 out]
    n204 = shared-variable "RT CompactRIO Target\\Mod6\\DIO7"() -> (w482:bool)  [unwired: 1 in, 1 out]
    n205 = shared-variable "RT CompactRIO Target\\Mod6\\DIO6"() -> (w481:bool)  [unwired: 1 in, 1 out]
    n206 = shared-variable "RT CompactRIO Target\\Mod6\\DIO5"() -> (w480:bool)  [unwired: 1 in, 1 out]
    n207 = shared-variable "RT CompactRIO Target\\Mod6\\DIO4"() -> (w479:bool)  [unwired: 1 in, 1 out]
    n208 = shared-variable "RT CompactRIO Target\\Mod6\\DIO3"() -> (w478:bool)  [unwired: 1 in, 1 out]
    n209 = shared-variable "RT CompactRIO Target\\Mod6\\DIO2"() -> (w477:bool)  [unwired: 1 in, 1 out]
    n210 = shared-variable "RT CompactRIO Target\\Mod6\\DIO1"() -> (w476:bool)  [unwired: 1 in, 1 out]
    n211 = shared-variable "RT CompactRIO Target\\Mod6\\DIO0"() -> (w475:bool)  [unwired: 1 in, 1 out]
    n212 = Bundle By Name(cluster=T9 {"MSB"=FALSE, "13th bit"=FALSE, "12th bit"=FALSE, "11th bit"=FALSE, "10th bit"=FALSE, "9th bit"=FALSE, "8th bit"=FALSE, "7th bit"=FALSE, "6th bit"=FALSE, "5th bit"=FALSE, "4th bit"=FALSE, "3rd bit"=FALSE, "2nd bit"=FALSE, "LSB"=FALSE} ("Cluster"), "MSB"=w488, "13th bit"=w487, "12th bit"=w486, "11th bit"=w485, "10th bit"=w484, "9th bit"=w483, "8th bit"=w482, "7th bit"=w481, "6th bit"=w480, "5th bit"=w479, "4th bit"=w478, "3rd bit"=w477, "2nd bit"=w476, "LSB"=w475) -> (w473:T9)
    n213 = call "Encoder-Decoder.vi"("Encoder data"=w473) -> ("Raw bits"=w490:bool[], "Converted bits"=w492:bool[], "Encoder position"=w491:u16)  [unwired: 8 in]
    "Encoder Position" <- w491
    "Encoder rotation" <- w491
    "Raw Encoder" <- w490
    "Converted Encoder" <- w492
    n214 = shared-variable "RT CompactRIO Target\\SCB shared var.lvlib\\SCB Encoder Position"(w491) -> ()  [unwired: 1 in, 1 out]
    n215 = shared-variable "RT CompactRIO Target\\SCB shared var.lvlib\\SCB Converted Encoder"(w492) -> ()  [unwired: 1 in, 1 out]
    n216 = shared-variable "RT CompactRIO Target\\SCB shared var.lvlib\\SCB Raw Encoder"(w490) -> ()  [unwired: 1 in, 1 out]
    n217 = local read "Stop"() -> (w472:bool)
    n218 = node-c288() -> ()  [unwired: 1 in, 1 out]
  }
  "Encoder readback" <- w4
  n219 = disable-structure shown="Disabled" {
    frame Disabled {
      w501 = 2 items=["Configuration Mode"=1, "Active Mode"=2] ("mode (Active Mode)")
      w503 = 1 items=["Configuration Mode"=1, "Active Mode"=2] ("mode (Active Mode)")
      n220 = property on="Motor status" class="Bool (strict)"("Value"=FALSE ("Motor status")) -> (error out=w495:errorcluster)  [unwired: 2 in, 1 out]
      n221 = property on="Stop" class="Bool (strict)"(error in=w495, "Value"=FALSE ("Stop")) -> (error out=w497:errorcluster)  [unwired: 1 in, 1 out]
      n222 = call <vilib>:"Set Scan Engine Mode.vi"("mode (Active Mode)"=w503, "error in (no error)"=w497) -> ("error out"=w500:errorcluster)  [unwired: 13 in]
      n223 = call <vilib>:"Clear All Faults.vi"("error in (no error)"=w500) -> ("error out"=w507:errorcluster)  [unwired: 10 in]
      n224 = call <vilib>:"Initialize Session.vi"("error in (no error)"=w507) -> ("error out"=w508:errorcluster, "Session out"=w509:refnum<k21>)  [unwired: 9 in]
      n225 = call-poly <vilib>:"Find.vi"("error in (no error)"=w508, "Experts"="mcSysApi" ("experts"), "Session in"=w509) -> ("error out"=w499:errorcluster, "Resources out"=w505:refnum<k20>[])  [unwired: 5 in, 2 out]
      n226 = Index Array(array=w505) -> (element=w506:refnum<k20>)  [unwired: 1 in]
      n227 = call <vilib>:"Reset Resource.vi"("error in (no error)"=w499, "Resource in"=w506) -> ("error out"=w502:errorcluster)  [unwired: 6 in, 3 out]
      n228 = call <vilib>:"Set Scan Engine Mode.vi"("mode (Active Mode)"=w501, "error in (no error)"=w502) -> ()  [unwired: 13 in, 1 out]
    }
    frame Enabled {
    }
  }
  n229 = while {
    tunnel: w3 -> [w511]
    stop <- w510 stop-if-true
    # "Start Sample Change monitor -  checks shared variables from SC controller/monitor VIs"
    n230 = shared-variable "RT CompactRIO Target\\SCB shared var.lvlib\\SCB Encoder Offset"(error in=w511) -> (w517:i16, error out=w516:errorcluster)
    n231 = shared-variable "RT CompactRIO Target\\SCB shared var.lvlib\\SCB Random Change"(error in=w516) -> (w514:bool, error out=w515:errorcluster)
    n232 = shared-variable "RT CompactRIO Target\\SCB shared var.lvlib\\SCB Start Sample Change"(error in=w515) -> (w519:bool, error out=w512:errorcluster)
    n233 = shared-variable "RT CompactRIO Target\\SCB shared var.lvlib\\SCB Encoder radius"(error in=w512) -> (w513:i32)  [unwired: 1 out]
    n234 = local write "Random Sample"(w514) -> ()
    n235 = local write "Encoder offset"(w517) -> ()
    n236 = local write "Step Window radius"(w513) -> ()
    n237 = case shown="True" w519 {
      frame False {
      }
      frame True {
        n238 = shared-variable "RT CompactRIO Target\\SCB shared var.lvlib\\SCB Requested Sample"() -> (w522:u8)  [unwired: 1 in, 1 out]
        n239 = shared-variable "RT CompactRIO Target\\SCB shared var.lvlib\\SCB Start Sample Change"(FALSE ("Start Sample Change")) -> ()  [unwired: 1 in, 1 out]
        n240 = local write "Start Sample Change"(TRUE ("Start Sample Change")) -> ()
        n241 = local write "New Sample"(w522) -> ()
        n242 = local write "Current State"(SC2_states."change sample" ("Current State")) -> ()
      }
    }
    n243 = local read "Stop"() -> (w510:bool)
    n244 = Wait Until Next ms Multiple(millisecond multiple=500) -> ()  [unwired: 1 out]
  }
  n245 = node-c288(w9) -> ()  [unwired: 1 out]
  n246 = while {
    stop <- FALSE stop-if-true
    # "Bypass Cluster Monitor"
    n247 = shared-variable "RT CompactRIO Target\\SCB shared var.lvlib\\SCB Bypass Control"() -> (w529:T10)  [unwired: 1 in, 1 out]
    n248 = Unbundle By Name(w529) -> ("SCB Insert Rod Bypass"=→"SCB Insert Rod Bypass":bool, "SCB Retract Rod Bypass"=→"SCB Retract Rod Bypass":bool, "SCB Sample Rod Bypass"=→"SCB Sample Rod Bypass":bool, "SCB Ion Source GV Bypass"=→"SCB Ion Source GV Bypass":bool, "SCB Wheel GV Bypass"=→"SCB Wheel GV Bypass":bool)
    n249 = Wait Until Next ms Multiple(millisecond multiple=u32 1000) -> ()  [unwired: 1 out]
  }
  n250 = while {
    stop <- FALSE stop-if-true
    # "Device Status Monitor Cluster"
    n251 = shared-variable "RT CompactRIO Target\\Mod7\\Insert Rod In"() -> (w571:bool)  [unwired: 1 in, 1 out]
    n252 = shared-variable "RT CompactRIO Target\\Mod7\\Insert Rod Out"() -> (w568:bool)  [unwired: 1 in, 1 out]
    n253 = shared-variable "RT CompactRIO Target\\Mod7\\Retract Rod In"() -> (w563:bool)  [unwired: 1 in, 1 out]
    n254 = shared-variable "RT CompactRIO Target\\Mod7\\Retract Rod Out"() -> (w560:bool)  [unwired: 1 in, 1 out]
    n255 = shared-variable "RT CompactRIO Target\\Mod7\\Sample Rod Down"() -> (w555:bool)  [unwired: 1 in, 1 out]
    n256 = shared-variable "RT CompactRIO Target\\Mod7\\Sample Rod Up"() -> (w553:bool)  [unwired: 1 in, 1 out]
    n257 = shared-variable "RT CompactRIO Target\\Mod7\\Ion Source GV open"() -> (w542:bool)  [unwired: 1 in, 1 out]
    n258 = shared-variable "RT CompactRIO Target\\Mod7\\Ion Source GV close"() -> (w543:bool)  [unwired: 1 in, 1 out]
    n259 = shared-variable "RT CompactRIO Target\\Mod7\\Wheel GV open"() -> (w540:bool)  [unwired: 1 in, 1 out]
    n260 = shared-variable "RT CompactRIO Target\\Mod7\\Wheel GV close"() -> (w541:bool)  [unwired: 1 in, 1 out]
    n261 = Exclusive Or(1:w568, 2:w571) -> (0:w570:bool)
    n262 = Exclusive Or(1:w560, 2:w563) -> (0:w562:bool)
    n263 = Select(t=Horizontal_Rod_states."rod out", s=w568, f=Horizontal_Rod_states."rod in") -> (s? t:f=w565:T7)
    n264 = Select(t=Horizontal_Rod_states."rod out", s=w560, f=Horizontal_Rod_states."rod in") -> (s? t:f=w557:T7)
    n265 = Exclusive Or(1:w553, 2:w555) -> (0:w554:bool)
    n266 = Select(t=Vertical_Rod_states."rod up", s=w553, f=Vertical_Rod_states."rod down") -> (s? t:f=w552:T6)
    n267 = Exclusive Or(1:w543, 2:w542) -> (0:w547:bool)
    n268 = Select(t=GV_states."closed", s=w543, f=GV_states."open") -> (s? t:f=w546:T5)
    n269 = Exclusive Or(1:w541, 2:w540) -> (0:w545:bool)
    n270 = Select(t=GV_states."closed", s=w541, f=GV_states."open") -> (s? t:f=w544:T5)
    n271 = Select(t=Horizontal_Rod_states."status unclear", s=w570, f=w565) -> (s? t:f=w564:T7)
    n272 = Select(t=Horizontal_Rod_states."status unclear", s=w562, f=w557) -> (s? t:f=w556:T7)
    n273 = Select(t=Vertical_Rod_states."status unclear", s=w554, f=w552) -> (s? t:f=w551:T6)
    n274 = Select(t=GV_states."status unclear", s=w547, f=w546) -> (s? t:f=w535:T5)
    n275 = Select(t=GV_states."status unclear", s=w545, f=w544) -> (s? t:f=w536:T5)
    n276 = shared-variable "RT CompactRIO Target\\SCB shared var.lvlib\\SCB Ion Source GV Status"(w536) -> ()  [unwired: 1 in, 1 out]
    n277 = shared-variable "RT CompactRIO Target\\SCB shared var.lvlib\\SCB Sample Rod Status"(w551) -> ()  [unwired: 1 in, 1 out]
    n278 = shared-variable "RT CompactRIO Target\\SCB shared var.lvlib\\SCB Retract Rod Status"(w556) -> ()  [unwired: 1 in, 1 out]
    n279 = shared-variable "RT CompactRIO Target\\SCB shared var.lvlib\\SCB Insert Rod Status"(w564) -> ()  [unwired: 1 in, 1 out]
    n280 = shared-variable "RT CompactRIO Target\\SCB shared var.lvlib\\SCB Wheel GV Status"(w535) -> ()  [unwired: 1 in, 1 out]
    n281 = Wait Until Next ms Multiple(millisecond multiple=u32 100) -> ()  [unwired: 1 out]
  }
  n282 = node-c288(w7) -> ()  [unwired: 1 out]
